vi "LEDModeController.vi"(9 "Locate LED":bool, 10 "Choose Hue":bool) -> (2 "LED Mode":T1(ring))   [LabVIEW 2019]
uses:
  dsdata.vi
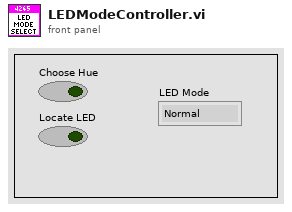
[diagram p1: front panel]
types:
  T1 = enum16{"Normal", "Party Mode", "Choose Hue", "Debug", "Locate LED"}
  T2 = typedef "WPI_DriverStationRobotMode2.ctl" = enum16{"Autonomous Disabled", "Autonomous Enabled", "Teleop Disabled", "Teleop Enabled", "Disconnected", "Finish", "Test Disabled", "Test Enabled", "Emergency Stopped"}
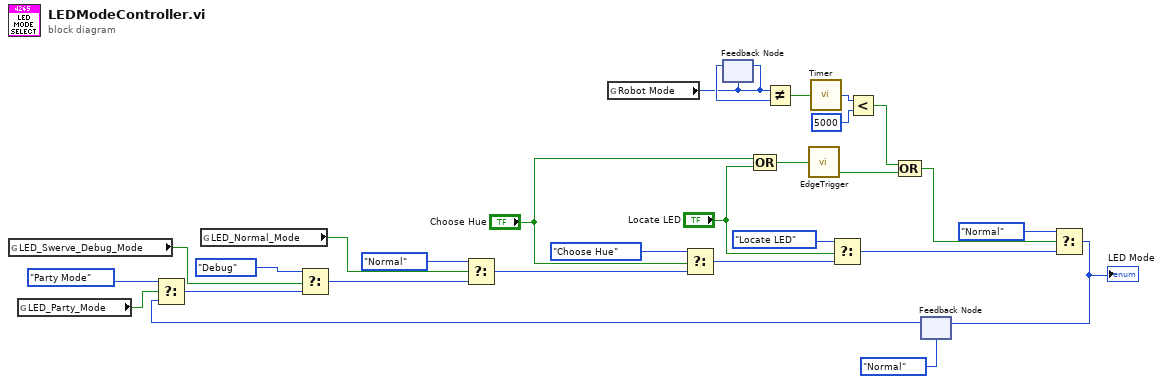
[diagram p0: block diagram]
diagram:
  n1 = global read "dsdata.vi" "LED_Swerve_Debug_Mode"() -> (w5:bool)
  n2 = global read "dsdata.vi" "LED_Party_Mode"() -> (w6:bool)
  n3 = global read "dsdata.vi" "LED_Normal_Mode"() -> (w3:bool)
  n4 = global read "dsdata.vi" "Robot Mode"() -> (w27:T2)
  n5 = feedback #1(w27) -> (w28:T2)
  n6 = feedback-in #1(w27) -> ()
  n7 = Compound Arithmetic op=OR("Choose Hue", "Locate LED") -> (w9:bool)
  n8 = Not Equal?(x=w27, y=w28) -> (x != y?=w26:bool)
  n9 = call "EdgeTrigger.vi"("Input Signal"=w9) -> ("Falling Edge Trigger"=w8:bool)  [unwired: 2 out]
  n10 = call "Timer.vi"("Reset Timer"=w26) -> ("Time (ms)"=w19:u32)
  n11 = Less?(x=w19, y=u32 5000) -> (x < y?=w17:bool)
  n12 = Compound Arithmetic op=OR(w17, w8) -> (w16:bool)
  n13 = feedback #2(T1."Normal") -> (w13:T1)
  n14 = Select(t=T1."Party Mode", s=w6, f=w13) -> (s? t:f=w24:T1)
  n15 = Select(t=T1."Debug", s=w5, f=w24) -> (s? t:f=w2:T1)
  n16 = Select(t=T1."Normal", s=w3, f=w2) -> (s? t:f=w1:T1)
  n17 = Select(t=T1."Choose Hue", s="Choose Hue", f=w1) -> (s? t:f=w20:T1)
  n18 = Select(t=T1."Locate LED", s="Locate LED", f=w20) -> (s? t:f=w15:T1)
  n19 = Select(t=T1."Normal", s=w16, f=w15) -> (s? t:f=w7:T1)
  "LED Mode" <- w7
  n20 = feedback-in #2(w7) -> ()
